vi "Protection_function_R2.vi"(4 "Transfer Trip":bool, 5 "RMS minimum\nvalues":cluster{"VRMS values":dbl, "IRMS values":dbl}, 6 "Blocking in":bool, 7 "Reset Relay":bool, 8 "input cluster":T3, 9 "Total power values":dbl[](array[numeric]), 10 "RMS values":dbl[](array[numeric]), 11 "Protection settings":T4) -> (0 "output cluster":T3, 1 "Blocking out":bool[](array[boolean]), 2 "Reclose":bool, 3 "trip signal":bool)   [LabVIEW 2016]
uses:
  <vilib>/addons/Electrical Power/Protection/Definite Time Delay/subVIs/fpga_Timer Feedback Var.ctl
  <vilib>/addons/Electrical Power/Protection/Definite Time Delay/subVIs/fpga_State.ctl
  <vilib>/addons/Electrical Power/Protection/Inverse Time Delay/subVIs/ep_Operate Time.ctl
  <vilib>/addons/Electrical Power/Protection/NI_EP_Protection.lvlib
  <vilib>/addons/Electrical Power/Protection/NI_EP_Protection_FPGA.lvlib
panel:
  out "VR error":i32
  out "I error":i32
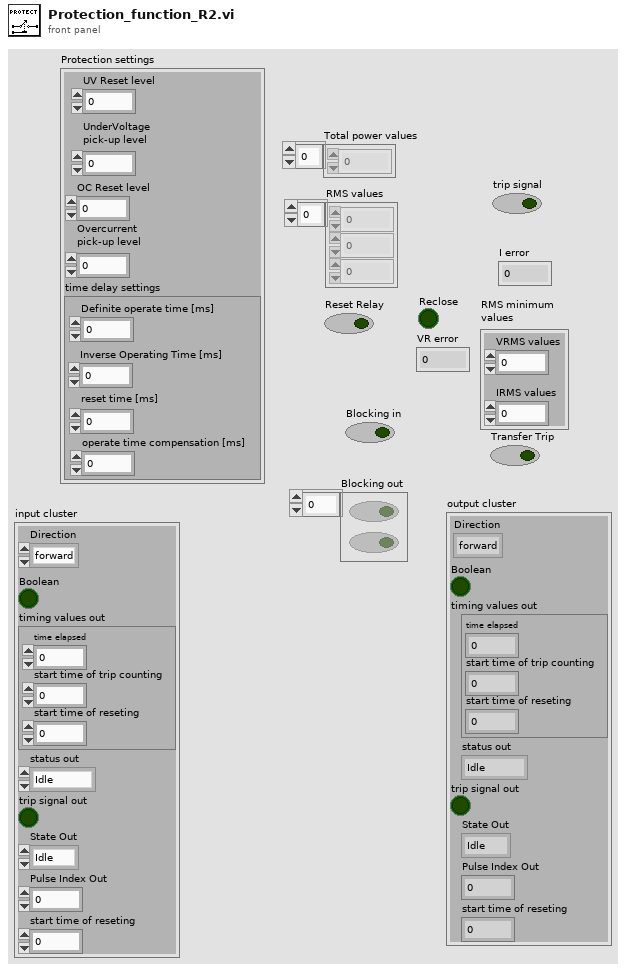
[diagram p1: front panel]
types:
  T1 = typedef "NI_EP_Protection_FPGA.lvlib/fpga_Timer Feedback Var.ctl" = cluster{"time elapsed":u32, "start time of trip counting":u32, "start time of reseting":u32}
  T2 = typedef "NI_EP_Protection_FPGA.lvlib/fpga_State.ctl" = enum16{"Idle", "Trip Counting", "Tripped", "Reset Counting"}
  T3 = cluster{"Direction":enum16{"forward", "backward", "N/D"}, "Boolean":bool, "timing values out":T1, "status out":T2, "trip signal out":bool, "State Out":enum16{"Idle", "Wait for Trip", "PulseClosing", "Locked"}, "Pulse Index Out":i32, "start time of reseting":u32}
  T4 = cluster{"UV Reset level":dbl, "UnderVoltage \npick-up level":dbl, "OC Reset level":dbl, "Overcurrent\npick-up level":dbl, "time delay settings":cluster{"Definite operate time [ms]":u32, "Inverse Operating Time [ms]":u32, "reset time [ms]":u32, "operate time compensation [ms]":u32}}
  T5 = enum16{"Idle", "Wait for Trip", "PulseClosing", "Locked"}
  T6 = cluster{"Definite operate time [ms]":u32, "Inverse Operating Time [ms]":u32, "reset time [ms]":u32, "operate time compensation [ms]":u32}
  T7 = typedef "NI_EP_Protection.lvlib/ep_Operate Time.ctl" = cluster{"A [s]":dbl, "B [s]":dbl, "alpha":dbl, "K2 [s]":dbl, "K1 [s]":dbl, "K3 [s]":dbl}
  T8 = cluster{u32, "reset time [ms]":u32, "reset time [ms]":u32}
  T9 = cluster{"Definite operate time [ms]":u32, "reset time [ms]":u32, "reset time [ms]":u32}
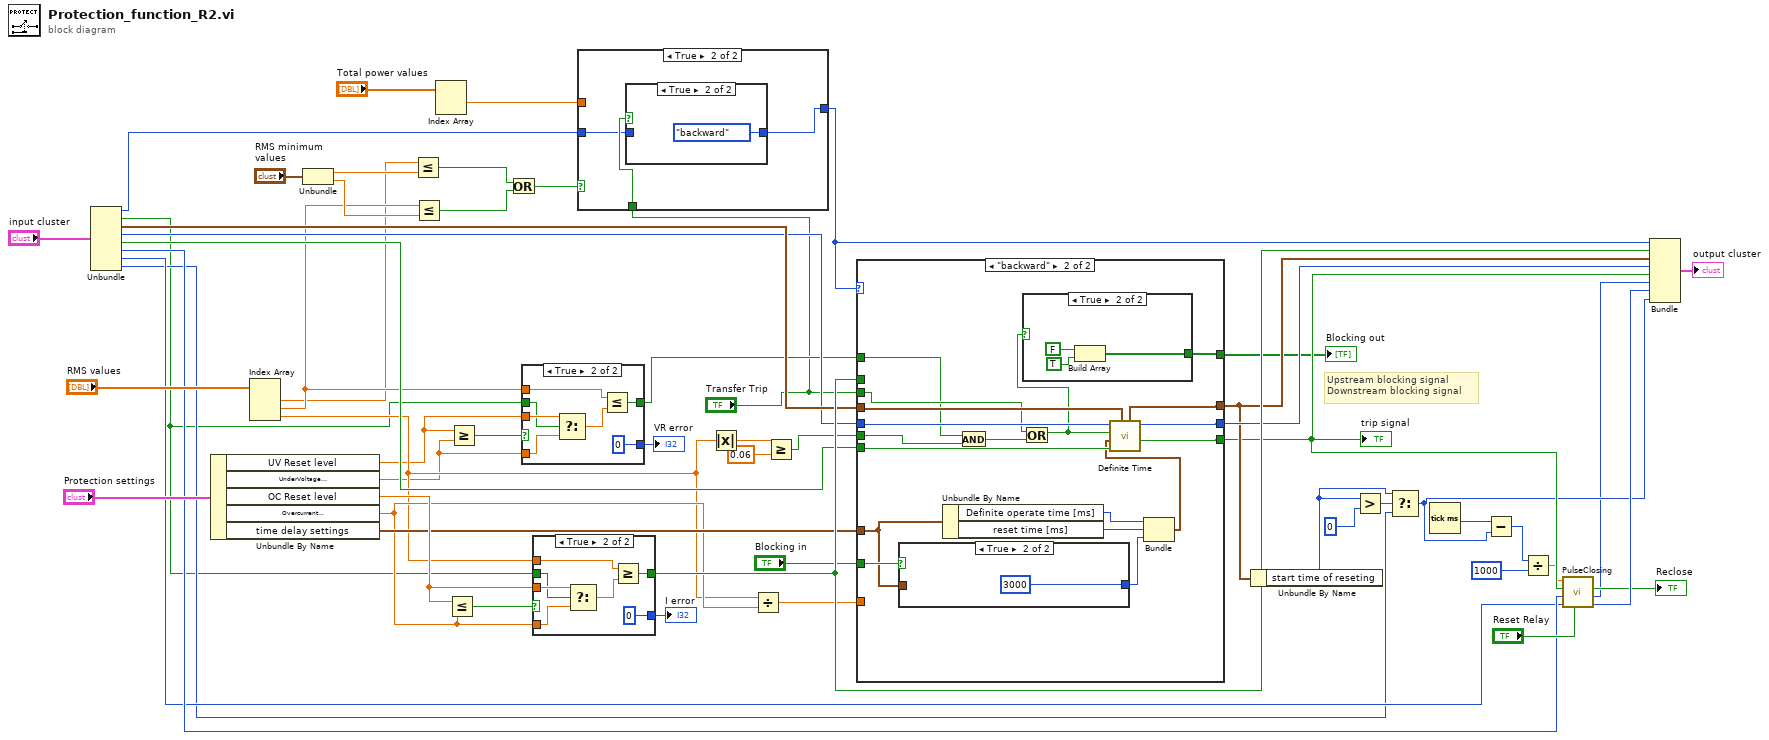
[diagram p0: block diagram]
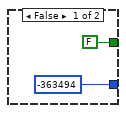
[diagram p2: hidden frame]
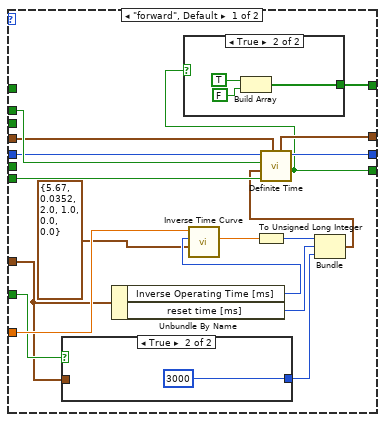
[diagram p3: hidden frame]
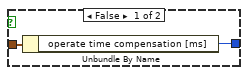
[diagram p4: hidden frame]
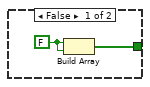
[diagram p5: hidden frame]
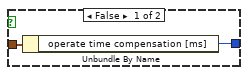
[diagram p6: hidden frame]
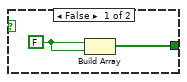
[diagram p7: hidden frame]
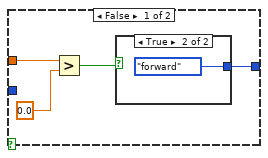
[diagram p8: hidden frame]
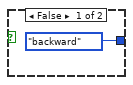
[diagram p9: hidden frame]
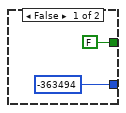
[diagram p11: hidden frame]
diagram:
  # "Upstream blocking signal\nDownstream blocking signal"
  n1 = Unbundle("input cluster") -> ("Direction"=w31:enum16{"forward", "backward", "N/D"}, "Boolean"=w1:bool, "timing values out"=w18:T1, "status out"=w17:T2, "trip signal out"=w16:bool, "State Out"=w15:T5, "Pulse Index Out"=w14:i32, "start time of reseting"=w13:u32)
  n2 = Unbundle By Name("Protection settings") -> ("UV Reset level"=w4:dbl, "UnderVoltage \npick-up level"=w3:dbl, "OC Reset level"=w49:dbl, "Overcurrent\npick-up level"=w34:dbl, "time delay settings"=w47:T6)
  n3 = Index Array(array="RMS values") -> (element #1=w5:dbl, element #2=w12:dbl, element #3=w10:dbl)  [unwired: 3 in]
  n4 = Unbundle("RMS minimum\nvalues") -> ("VRMS values"=w54:dbl, "IRMS values"=w51:dbl)
  n5 = Less Or Equal?(x=w5, y=w54) -> (x <= y?=w53:bool)
  n6 = Less Or Equal?(x=w12, y=w51) -> (x <= y?=w52:bool)
  n7 = Index Array(array="Total power values") -> (element #1=w39:dbl)  [unwired: 2 in, 1 out]
  n8 = Less Or Equal?(x=w49, y=w34) -> (x <= y?=w57:bool)
  n9 = Greater Or Equal?(x=w4, y=w3) -> (x >= y?=w2:bool)
  n10 = Or(x=w53, y=w52) -> (x .or. y?=w44:bool)
  n11 = case shown="True" w2 {
    tunnel: [-363494 ("error") 0 ("error")] -> w20
    tunnel: w4 -> [_ w64]
    tunnel: w3 -> [_ w63]
    tunnel: [FALSE ("Boolean") w62] -> w11
    tunnel: w1 -> [_ w61]
    tunnel: w12 -> [_ w60]
    frame False {
    }
    frame True {
      n12 = Select(t=w64, s=w61, f=w63) -> (s? t:f=w66:dbl)
      n13 = Less Or Equal?(x=w60, y=w66) -> (x <= y?=w62:bool)
    }
  }
  "VR error" <- w20
  n14 = case shown="True" w57 {
    tunnel: [-363494 ("error") 0 ("error")] -> w56
    tunnel: w49 -> [_ w73]
    tunnel: w34 -> [_ w72]
    tunnel: [FALSE ("Boolean") w71] -> w48
    tunnel: w1 -> [_ w70]
    tunnel: w10 -> [_ w69]
    frame False {
    }
    frame True {
      n15 = Select(t=w73, s=w70, f=w72) -> (s? t:f=w75:dbl)
      n16 = Greater Or Equal?(x=w69, y=w75) -> (x >= y?=w71:bool)
    }
  }
  "I error" <- w56
  n17 = case shown="True" w44 {
    tunnel: w39 -> [w77 _]
    tunnel: w31 -> [_ w82]
    tunnel: [w76 w83] -> w30
    tunnel: "Transfer Trip" -> [_ w84]
    frame False {
      n18 = Greater?(x=w77, y=0.0) -> (0:w78:bool)
      n19 = case shown="True" w78 {
        tunnel: [enum16{"forward", "backward"}."backward" enum16{"forward", "backward"}."forward"] -> w76
        frame False {
        }
        frame True {
        }
      }
    }
    frame True {
      n20 = case shown="True" w84 {
        tunnel: [w85 enum16{"forward", "backward", "N/D"}."backward" ("Direction")] -> w83
        tunnel: w82 -> [w85 _]
        frame False {
        }
        frame True {
        }
      }
    }
  }
  n21 = Absolute Value(x=w10) -> (abs(x)=w6:dbl)
  n22 = Divide(x=w10, y=w34) -> (x/y=w45:dbl)
  n23 = Greater Or Equal?(x=w6, y=0.06) -> (x >= y?=w8:bool)
  n24 = case shown="\"backward\"" w30 {
    tunnel: w48 -> [w104 _]
    tunnel: w47 -> [w88 w120]
    tunnel: [w103 w125] -> w46
    tunnel: w45 -> [w102 _]
    tunnel: [w101 w126] -> w43
    tunnel: [w100 w124] -> w35
    tunnel: w18 -> [w99 w129]
    tunnel: w17 -> [w98 w128]
    tunnel: w16 -> [w97 w127]
    tunnel: [w90 w123] -> w22
    tunnel: "Blocking in" -> [w89 w122]
    tunnel: w8 -> [_ w113]
    tunnel: w11 -> [_ w115]
    tunnel: "Transfer Trip" -> [_ w117]
    frame "forward", Default {
      n25 = case shown="True" w89 {
        tunnel: [w105 u32 3000 ("reset time [ms]")] -> w87
        tunnel: w88 -> [w106 _]
        frame False {
          n26 = Unbundle By Name(w106) -> ("operate time compensation [ms]"=w105:u32)
        }
        frame True {
        }
      }
      n27 = Unbundle By Name(w88) -> ("Inverse Operating Time [ms]"=w96:u32, "reset time [ms]"=w93:u32)
      n28 = call "Inverse Time Curve.vi"("input cluster"=T7 {"A [s]"=5.67, "B [s]"=0.0352, "alpha"=2.0, "K2 [s]"=1.0, "K1 [s]"=0.0, "K3 [s]"=0.0}, "time dial"=w96, "multiples of pickup"=w102) -> ("original time"=w94:dbl)  [unwired: 5 in, 1 out]
      n29 = To Unsigned Long Integer(number=w94) -> (unsigned 32bit integer=w91:u32)
      n30 = Bundle(w91, "reset time [ms]"=w93, "reset time [ms]"=w87) -> (w92:T8)  [unwired: 1 in]
      n31 = call "Definite Time.vi"("timing values in"=w99, "trip signal in"=w97, "time delay settings"=w92, "pick-up signal? (F)"=w104, "status in"=w98) -> ("trip signal out"=w100:bool, "status out"=w103:T2, "timing values out"=w101:T1)  [unwired: 3 in, 1 out]
      n32 = case shown="True" w100 {
        tunnel: [w108 w110] -> w90
        frame False {
          w109 = FALSE
          n33 = Build Array(w109, w109) -> (w108:bool[])
        }
        frame True {
          n34 = Build Array(TRUE, FALSE) -> (w110:bool[])
        }
      }
    }
    frame "backward" {
      n35 = case shown="True" w122 {
        tunnel: [w131 u32 3000 ("reset time [ms]")] -> w121
        tunnel: w120 -> [w132 _]
        frame False {
          n36 = Unbundle By Name(w132) -> ("operate time compensation [ms]"=w131:u32)
        }
        frame True {
        }
      }
      n37 = Unbundle By Name(w120) -> ("Definite operate time [ms]"=w119:u32, "reset time [ms]"=w130:u32)
      n38 = And(x=w115, y=w113) -> (x .and. y?=w114:bool)
      n39 = Or(x=w117, y=w114) -> (x .or. y?=w116:bool)
      n40 = case shown="True" w116 {
        tunnel: [w134 w136] -> w123
        frame False {
          w135 = FALSE
          n41 = Build Array(w135, w135) -> (w134:bool[])
        }
        frame True {
          n42 = Build Array(FALSE, TRUE) -> (w136:bool[])
        }
      }
      n43 = Bundle("Definite operate time [ms]"=w119, "reset time [ms]"=w130, "reset time [ms]"=w121) -> (w118:T9)  [unwired: 1 in]
      n44 = call "Definite Time.vi"("timing values in"=w129, "trip signal in"=w127, "time delay settings"=w118, "pick-up signal? (F)"=w116, "status in"=w128) -> ("trip signal out"=w124:bool, "status out"=w125:T2, "timing values out"=w126:T1)  [unwired: 3 in, 1 out]
    }
  }
  "trip signal" <- w35
  "Blocking out" <- w22
  n45 = Unbundle By Name(w43) -> ("start time of reseting"=w27:u32)
  n46 = Greater?(x=w27, y=u32 0 ("x")) -> (0:w28:bool)
  n47 = Select(t=w27, s=w28, f=w13) -> (s? t:f=w26:u32)
  n48 = Tick Count (ms)() -> (millisecond timer value=w42:u32)
  n49 = Subtract(x=w42, y=w26) -> (x-y=w37:u32)
  n50 = Divide(x=w37, y=u32 1000) -> (x/y=w25:dbl)
  n51 = call "PulseClosing.vi"("Reset Relay"="Reset Relay", "Pulse Index In"=w14, "State In"=w15, "Trip signal"=w35, "Time lapsed"=w25) -> ("Pulse Index Out"=w36:i32, "State Out"=w24:T5, "Reclose"=→"Reclose":bool)  [unwired: 4 in]
  n52 = Bundle("Direction"=w30, "Boolean"=w48, "timing values out"=w43, "status out"=w46, "trip signal out"=w35, "State Out"=w24, "Pulse Index Out"=w36, "start time of reseting"=w26) -> (→"output cluster":T3)  [unwired: 1 in]
